vi "DataIn.vi"() -> (5 "Array Head":i16, 7 "ArrayAnalogIn 0":i16[](array[numeric]), 8 "ArrayAnalogIn 1":i16[](array[numeric]), 9 "ArrayAnalogIn 2":i16[](array[numeric]), 10 "ArrayAnalogIn 3":i16[](array[numeric]))   [LabVIEW 2020]
uses:
  <vilib>/eio/EIONode/EIONode.xnode
  <vilib>/rvi/eio/common/nirviEmuTemplateMethod_errors.vi
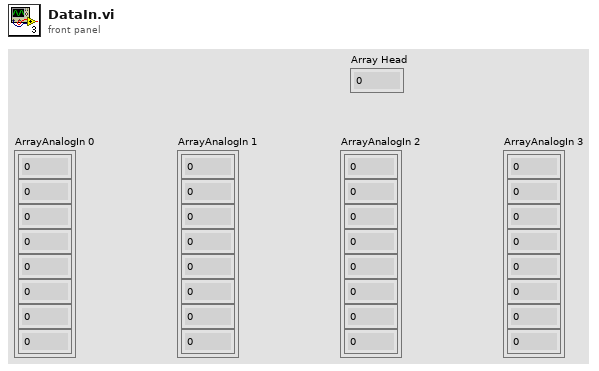
[diagram p1: front panel]
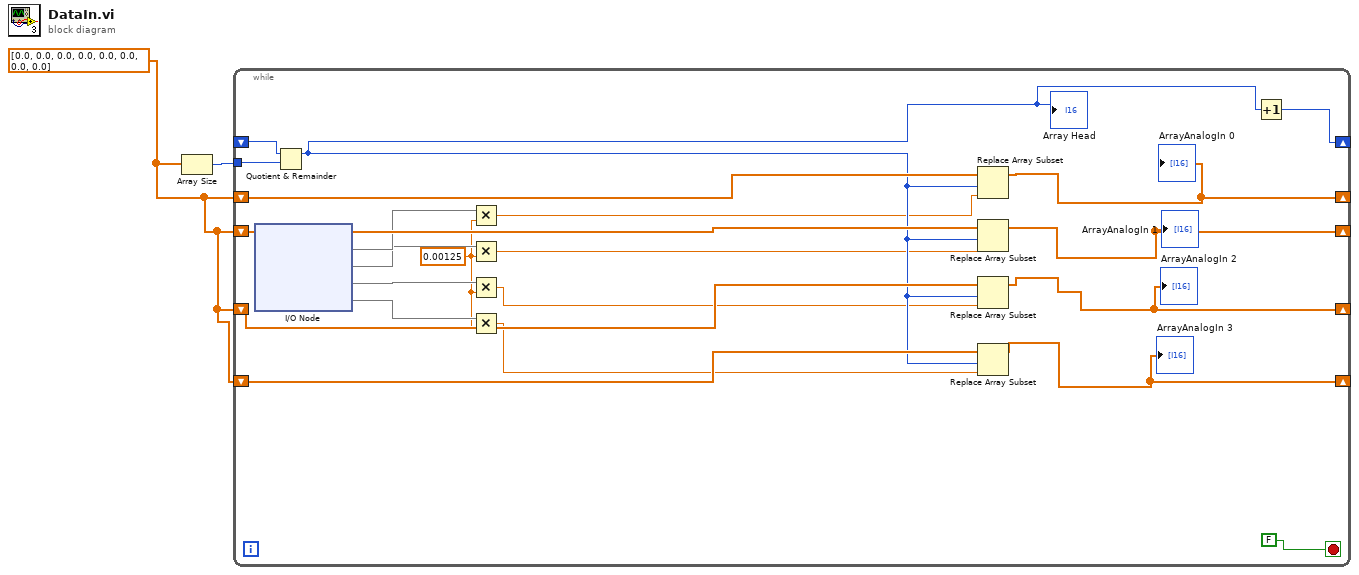
[diagram p0: block diagram]
diagram:
  w1 = dbl[] [0.0, 0.0, 0.0, 0.0, 0.0, 0.0, 0.0, 0.0]
  n1 = Array Size(array=w1) -> (size(s)=w2:i32)
  n2 = while {
    shift-right: [w19] -> _
    shift-left: w1 -> [w24]
    shift-right: [w18] -> _
    shift-left: w1 -> [w23]
    shift-right: [w17] -> _
    shift-left: w1 -> [w22]
    shift-right: [w16] -> _
    shift-left: w1 -> [w21]
    shift-right: [w14] -> _
    shift-left: _ -> [w15]
    tunnel: w2 -> [w12]
    stop <- FALSE stop-if-true
    w3 = 0.00125
    n3 = xnode "I/O Node"() -> ("AnalogIn0"=w11, "AnalogIn1"=w9, "AnalogIn2"=w8, "AnalogIn3"=w7)  [unwired: 4 in, 4 out]
    n4 = Quotient & Remainder(x=w15, y=w12) -> (x-y*floor(x/y)=w13:i32)  [unwired: 1 out]
    "Array Head" <- w13
    n5 = Multiply(x=w11, y=w3) -> (x*y=w10:dbl)
    n6 = Multiply(x=w9, y=w3) -> (x*y=w4:dbl)
    n7 = Multiply(x=w8, y=w3) -> (x*y=w5:dbl)
    n8 = Multiply(x=w7, y=w3) -> (x*y=w6:dbl)
    n9 = Replace Array Subset(array=w24, new element=w10, index=w13) -> (w19:dbl[])
    "ArrayAnalogIn 0" <- w19
    n10 = Replace Array Subset(array=w23, new element=w4, index=w13) -> (w18:dbl[])
    "ArrayAnalogIn 1" <- w18
    n11 = Replace Array Subset(array=w22, new element=w5, index=w13) -> (w17:dbl[])
    "ArrayAnalogIn 2" <- w17
    n12 = Replace Array Subset(array=w21, new element=w6, index=w13) -> (w16:dbl[])
    "ArrayAnalogIn 3" <- w16
    n13 = Increment(x=w13) -> (x+1=w14:i32)
  }
